vi "sub_main_pid.vi"(8 "error in":errorcluster) -> (0 "error out":errorcluster)   [LabVIEW 2019]
uses:
  <vilib>/Platform/TimedLoop/XDataNode/timing_clust.ctl
  <vilib>/Platform/TimedLoop/XDataNode/nitl_modes.ctl
  <vilib>/Platform/TimedLoop/XDataNode/wakeup.ctl
  Ctrl/cmd_common.ctl
  Ctrl/pid-in-params.ctl
  Ctrl/gps-databuf.ctl
  <vilib>/addons/control/pid/pid.llb/PID (DBL).vi
  <vilib>/Platform/TimedLoop/XDataNode/XDataNode.xnode
  <vilib>/addons/control/pid/NI_PID_pid.lvlib
  <vilib>/Platform/TimedLoop/XDataNode/XDNodeRunTimeDep.lvlib
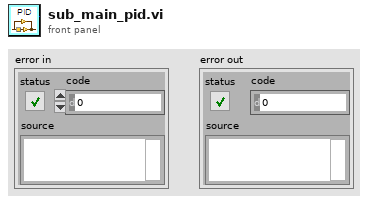
[diagram p1: front panel]
types:
  T1 = cluster{"PID gains":cluster{"proportional gain (Kc)":dbl, "integral time (Ti, min)":dbl, "derivative time (Td, min)":dbl}, "PID limits":cluster{"output high":dbl, "output low":dbl}, "dt_pid":u32}
  T2 = typedef "pid-in-params.ctl" = enum16{"read", "write"}
  T3 = typedef "gps-databuf.ctl" = enum16{"read", "write"}
  T4 = cluster{"rawdata":string, "GPS Data":cluster{"Latitude":cluster{"Valid?":bool, "Latitude (Deg)":dbl}, "Longitude":cluster{"Valid?":bool, "Longitude (Deg)":dbl}, "Height":cluster{"Valid?":bool, "Height (m)":dbl}, "Undulation":cluster{"Valid?":bool, "Undulation(m)":dbl}, "North Vel":cluster{"Valid?":bool, "North Vel (m/s)":dbl}, "East Vel":cluster{"Valid?":bool, "East Vel (m/s)":dbl}, "Up Vel":cluster{"Valid?":bool, "Up Vel (m/s)":dbl}, "Roll":cluster{"Valid?":bool, "Roll (degrees)":dbl}, "Pitch":cluster{"Valid?":bool, "Pitch (degrees)":dbl}, "Azimuth":cluster{"Valid?":bool, "Azimuth (degrees)":dbl}, "Lat deviation":cluster{"Valid?":bool, "Lat deviation (m)":dbl}, "Long deviation":cluster{"Valid?":bool, "Long deviation (m)":dbl}, "Height deviation":cluster{"Valid?":bool, "Height deviation (m)":dbl}, "North vel deviation":cluster{"Valid?":bool, "North vel deviation (m/s)":dbl}, "East vel deviation":cluster{"Valid?":bool, "East vel deviation (m/s)":dbl}, "Up vel deviation":cluster{"Valid?":bool, "Up vel deviation (m/s)":dbl}, "Roll deviation":cluster{"Valid?":bool, "Roll deviation (degrees)":dbl}, "Pitch deviation":cluster{"Valid?":bool, "Pitch deviation (degrees)":dbl}, "Azimuth deviation":cluster{"Valid?":bool, "Azimuth deviation (degrees)":dbl}, "Ext sol status":cluster{"Valid?":bool, "Ext sol status":dbl}}, "Heading":dbl, "utm-1":cluster{"XN":dbl, "YE":dbl}}
  T5 = cluster{"deg_agv-lookahead":dbl, "deg_waypoint":dbl, "deg_gap":dbl, "deg_target":dbl, "pid output":dbl, "dis-gap":dbl, "deg_agv-center":dbl}
  T6 = cluster{"proportional gain (Kc)":dbl, "integral time (Ti, min)":dbl, "derivative time (Td, min)":dbl}
  T7 = typedef "XDNodeRunTimeDep.lvlib/timing_clust.ctl" = cluster{"Expected End [f-1]":u64, "Actual End [f-1]":u64, "Finished Late? [f-1]":bool, "Expected End [i-1]":u64, "Actual End [i-1]":u64, "Finished Late? [i-1]":bool, "Expected Start [i]":u64, "Actual Start [i]":u64, "Expected Start [f]":u64, "Actual Start [f]":u64, "Source Name":string, "Structure Name":string, "Period":i64, "Deadline":i64, "Offset":i64, "Start":i64, "Priority":i32, "Timeout":i32, "Mode":T8, "Wakeup Reason":T9, "Error":errorcluster, "Source Type":string, "Secondary Source Type":string, "Global End Time":u64, "Global Start Time":u64, "Frame Duration":u64, "Iteration Duration":u64, "Assigned CPU":i32, "I/O Scan Engine Mode":u32}
  T8 = typedef "XDNodeRunTimeDep.lvlib/nitl_modes.ctl" = enum32{"No Change", "Process missed periods, maintain original phase", "Discard missed periods, maintain original phase", "Process missed periods, ignore original phase", "Discard missed periods, ignore original phase"}
  T9 = typedef "XDNodeRunTimeDep.lvlib/wakeup.ctl" = enum32{"Normal", "Aborted", "Asynchronous wakeup", "Timing source error", "Timed loop error", "Timeout"}
  T10 = typedef "cmd_common.ctl" = enum16{"read", "write"}
  T11 = typedef "joystick cfg.ctl" = cluster{"Type":enum16{"Logitech F710", "Xbox"}, "steer limit":cluster{"min":dbl, "max":dbl, "scale":dbl, "offset":dbl}, "speed limit":cluster{"min":dbl, "max":dbl, "pwm max":dbl}, "ID":i32, "joystick max":dbl}
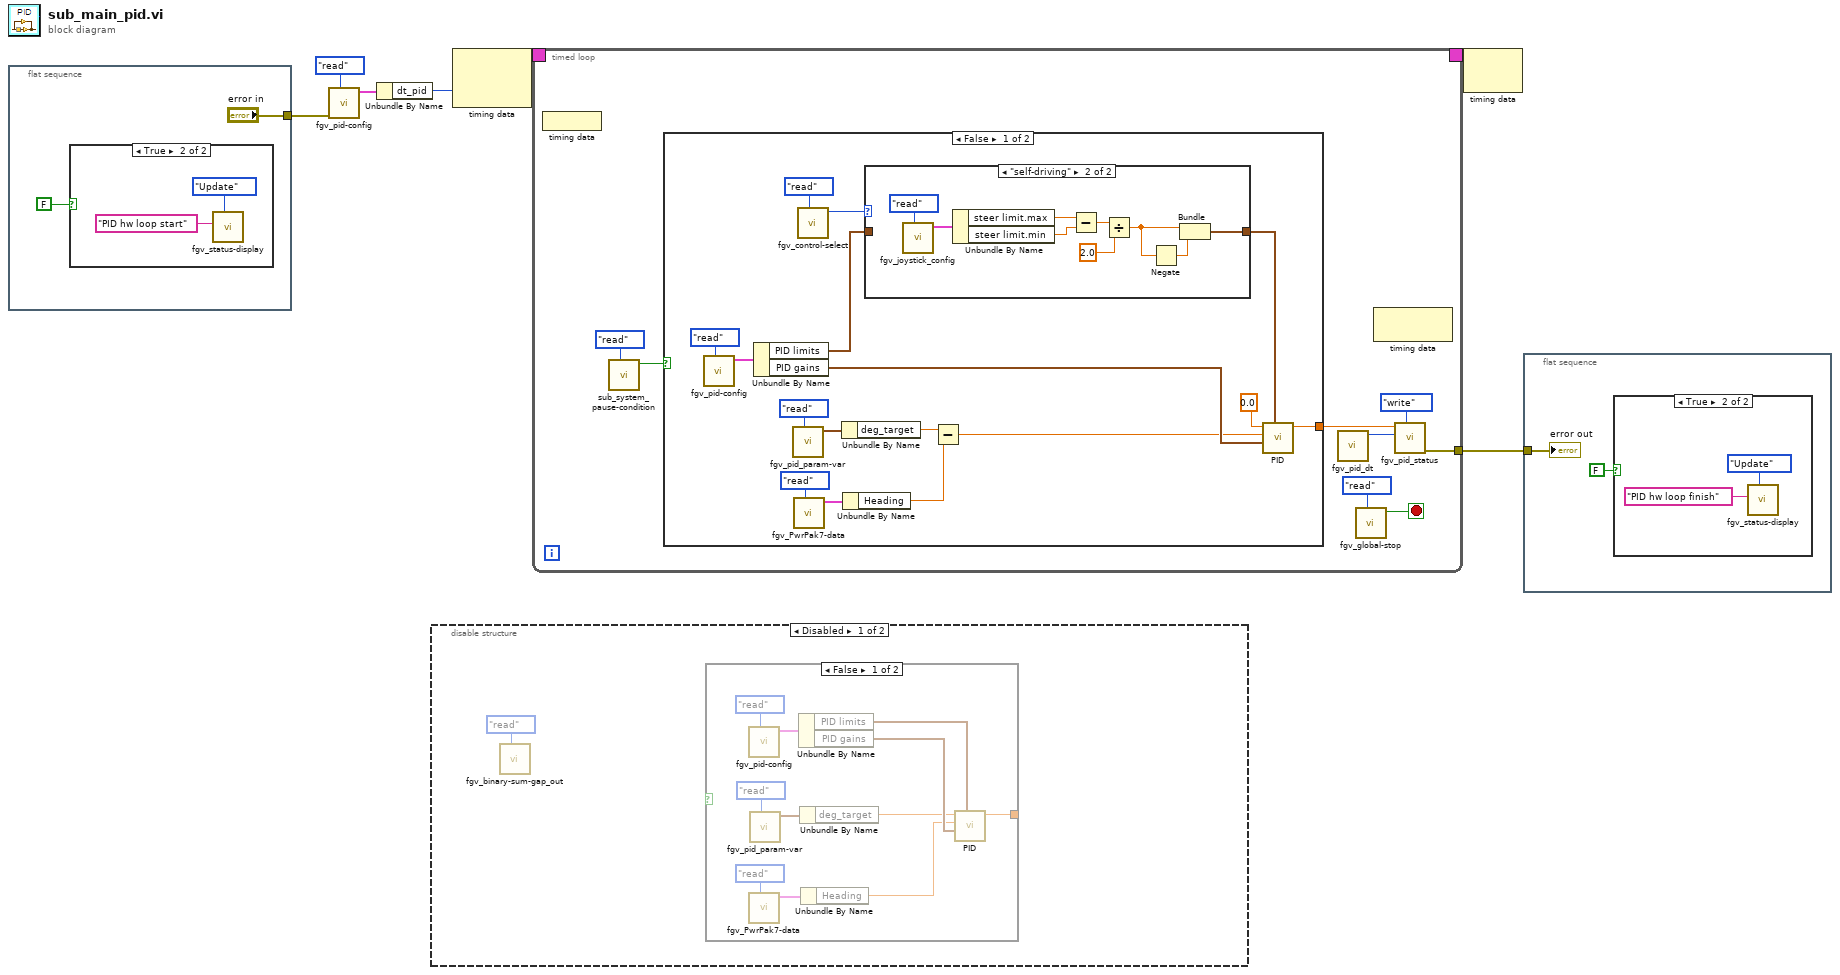
[diagram p0: block diagram]
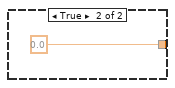
[diagram p2: hidden frame]
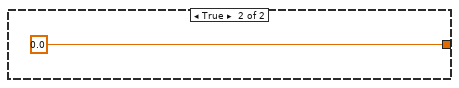
[diagram p7: hidden frame]
diagram:
  n1 = flat-sequence {
    tunnel: ["error in"] -> w3
    frame #0 {
      n2 = case shown="True" FALSE {
        frame False {
        }
        frame True {
          n3 = call "fgv_status-display.vi"("Mode"=enum16{"Initial", "Update", "Clear"}."Update", "title"="PID hw loop start" ("String in 1")) -> ()  [unwired: 9 in, 1 out]
        }
      }
    }
  }
  n4 = call "fgv_pid-config.vi"("cmd"=enum16{"read", "write"}."read", "error in"=w3) -> ("PID cfg out"=w2:T1)  [unwired: 8 in, 1 out]
  n5 = Unbundle By Name(w2) -> ("dt_pid"=w1:u32)
  n6 = disable-structure shown="Disabled" {
    frame Disabled {
      n7 = call "fgv_binary-sum-gap_out.vi"("cmd"=enum16{"read", "write"}."read") -> ()  [unwired: 10 in, 1 out]
      n8 = case shown="False" {
        selector: _ -> [_ _]
        tunnel: [w17 0.0] -> _
        frame False {
          n9 = call "fgv_pid-config.vi"("cmd"=enum16{"read", "write"}."read") -> ("PID cfg out"=w20:T1)  [unwired: 9 in, 1 out]
          n10 = call "fgv_PwrPak7-data.vi"("cmd"=gps-databuf."read") -> ("data cluster out"=w23:T4)  [unwired: 9 in, 1 out]
          n11 = call "fgv_pid_param-var.vi"("cmd"=pid-in-params."read") -> ("pid-var_output"=w15:T5)  [unwired: 10 in]
          n12 = Unbundle By Name(w20) -> ("PID limits"=w19:cluster{"output high":dbl, "output low":dbl}, "PID gains"=w18:T6)
          n13 = Unbundle By Name(w15) -> ("deg_target"=w14:dbl)
          n14 = Unbundle By Name(w23) -> ("Heading"=w13:dbl)
          n15 = call-poly <vilib>:"PID.vi"("output range"=w19, "PID gains"=w18, "process variable"=w13, "setpoint"=w14) -> ("output"=w17:dbl)  [unwired: 6 in, 1 out]
        }
        frame True {
        }
      }
    }
    frame Enabled {
    }
  }
  n16 = node-c288(w1) -> (w6:T7)  [unwired: 1 in]
  n17 = timed-loop {
    tunnel: [w27] -> w7
    timing: w6 -> [_]
    timing-out: [_] -> w5
    stop <- w30 stop-if-true
    n18 = node-c288() -> ()  [unwired: 1 in]
    n19 = call "sub_system_pause-condition.vi"("cmd"=enum16{"pause", "go", "read"}."read") -> ("pause"=w28:bool)  [unwired: 10 in]
    n20 = case shown="False" w28 {
      tunnel: [w45 0.0] -> w32
      frame False {
        n21 = call "fgv_pid-config.vi"("cmd"=enum16{"read", "write"}."read") -> ("PID cfg out"=w47:T1)  [unwired: 9 in, 1 out]
        n22 = Unbundle By Name(w47) -> ("PID limits"=w34:cluster{"output high":dbl, "output low":dbl}, "PID gains"=w46:T6)
        n23 = call "fgv_pid_param-var.vi"("cmd"=pid-in-params."read") -> ("pid-var_output"=w42:T5)  [unwired: 10 in]
        n24 = call "fgv_PwrPak7-data.vi"("cmd"=gps-databuf."read") -> ("data cluster out"=w40:T4)  [unwired: 9 in, 1 out]
        n25 = call "fgv_control-select.vi"("cmd"=cmd_common."read") -> ("mode out"=w35:enum16{"joystick", "self-driving"})  [unwired: 10 in]
        n26 = Unbundle By Name(w42) -> ("deg_target"=w39:dbl)
        n27 = Unbundle By Name(w40) -> ("Heading"=w38:dbl)
        n28 = case shown="\"self-driving\"" w35 {
          tunnel: w34 -> [w49 _]
          tunnel: [w49 w52] -> w33
          frame "joystick", Default {
          }
          frame "self-driving" {
            n29 = call "fgv_joystick_config.vi"("cmd"=cmd_common."read") -> ("Joystick cfg out"=w57:T11)  [unwired: 9 in, 1 out]
            n30 = Unbundle By Name(w57) -> ("steer limit.max"=w56:dbl, "steer limit.min"=w55:dbl)
            n31 = Subtract(x=w56, y=w55) -> (x-y=w54:dbl)
            n32 = Divide(x=w54, y=2.0) -> (x/y=w51:dbl)
            n33 = Negate(x=w51) -> (-x=w50:dbl)
            n34 = Bundle(w51, w50) -> (w52:cluster{dbl, dbl})  [unwired: 1 in]
          }
        }
        n35 = Subtract(x=w39, y=w38) -> (x-y=w37:dbl)
        n36 = call-poly <vilib>:"PID.vi"("output range"=w33, "PID gains"=w46, "process variable"=w37, "setpoint"=0.0) -> ("output"=w45:dbl)  [unwired: 6 in, 1 out]
      }
      frame True {
      }
    }
    n37 = call "fgv_pid_dt.vi"() -> ("ms"=w26:u32)  [unwired: 11 in]
    n38 = call "fgv_global-stop.vi"("cmd"=enum16{"init", "stop", "read"}."read") -> ("val_out"=w30:bool)  [unwired: 10 in]
    n39 = node-c288() -> ()  [unwired: 1 in, 1 out]
    n40 = call "fgv_pid_status.vi"("cmd"=cmd_common."write", "dt"=w26, "pid v"=w32) -> ("error out"=w27:errorcluster)  [unwired: 6 in, 2 out]
  }
  n41 = node-c288(w5) -> ()  [unwired: 1 out]
  n42 = flat-sequence {
    tunnel: w7 -> [w63]
    frame #0 {
      n43 = case shown="True" FALSE {
        frame False {
        }
        frame True {
          n44 = call "fgv_status-display.vi"("Mode"=enum16{"Initial", "Update", "Clear"}."Update", "title"="PID hw loop finish" ("String in 1")) -> ()  [unwired: 9 in, 1 out]
        }
      }
      "error out" <- w63
    }
  }
